vi "Speed.vi"(1 "Speed":dbl(knob) scale=1.0..6.0) -> (0 "x-y":dbl)   [LabVIEW 2021]
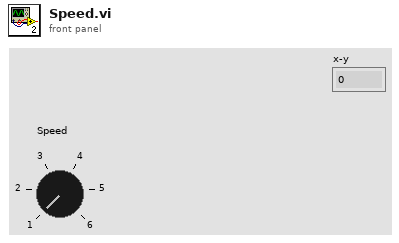
[diagram p1: front panel]
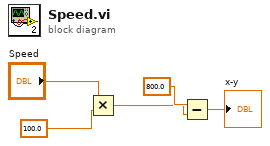
[diagram p0: block diagram]
diagram:
  n1 = Multiply(x="Speed", y=100.0 ("x*y")) -> (x*y=w2:dbl)
  n2 = Subtract(x=800.0, y=w2) -> (x-y=→"x-y":dbl)
